vi "ESA-C Set Voltage.vi"(2 "Voltage":dbl format="%.2f", 3 "Axis":i32, 4 "Drive Connection Settings":T1={"Objective GPIB-Port"=4, "Stage GPIB-Port"=4, "Drive Selector"=0, "Drive Velocity (V/s)"=5.0} {"Drive Velocity (V/s)" min=10.0 max=160.0 step=0.1 format="%.1f"; "Drive Selector" items=["Obj.", "Stage"]; "Stage GPIB-Port" min=1 max=20 step=1 format="%#.0f"; "Objective GPIB-Port" min=1 max=20 step=1 format="%#.0f"}) -> ()   [LabVIEW 2010]
uses:
  TypeDefs/ESA-C Connection Settings.ctl
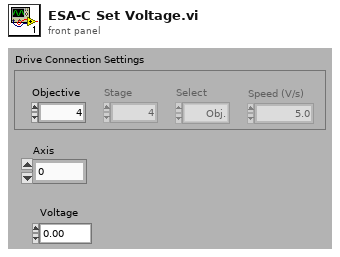
[diagram p1: front panel]
types:
  T1 = typedef "ESA-C Connection Settings.ctl" = cluster{"Objective GPIB-Port":i32, "Stage GPIB-Port":i32, "Drive Selector":u16, "Drive Velocity (V/s)":dbl}
  T2 = typedef "ESA-C Current Values.ctl" = cluster{"Voltages":cluster{"Drive X Voltage":dbl, "Drive Y Voltage":dbl, "Drive Z Voltage":dbl}, "Position":cluster{"Drive X Position":dbl, "Drive Y Position":dbl, "Drive Z Position":dbl}}
  T3 = cluster{"Drive X Voltage":dbl, "Drive Y Voltage":dbl, "Drive Z Voltage":dbl}
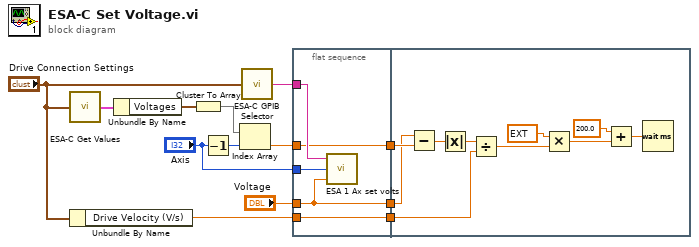
[diagram p0: block diagram]
diagram:
  n1 = call "ESA-C Get Values.vi"("Drive Connection Settings"="Drive Connection Settings") -> ("Drive Current Values"=w7:T2)
  n2 = Unbundle By Name("Drive Connection Settings") -> ("Drive Velocity (V/s)"=w3:dbl)
  n3 = Unbundle By Name(w7) -> ("Voltages"=w8:T3)
  n4 = Cluster To Array(cluster=w8) -> (array=w10:dbl[])
  n5 = Decrement(x="Axis") -> (x-1=w12:i32)
  n6 = Index Array(array=w10, index=w12) -> (element=w13:dbl)
  n7 = call "ESA-C GPIB Selector.vi"("Drive Connection Settings"="Drive Connection Settings") -> ("String"=w5:string)
  n8 = flat-sequence {
    tunnel: w5 -> [w18]
    tunnel: "Axis" -> [w17]
    tunnel: "Voltage" -> [w14]
    tunnel: w13 -> [w15]
    tunnel: [w16] -> w4
    tunnel: w3 -> [w16]
    tunnel: [w15] -> w2
    tunnel: [w14] -> w1
    tunnel: w4 -> [w23]
    tunnel: w2 -> [w20]
    tunnel: w1 -> [w19]
    frame #0 {
      n9 = call "ESA 1 Ax set volts.vi"("Voltage"=w14, "Axis"=w17, "GPIB Add"=w18) -> ()
    }
    frame #1 {
      n10 = Subtract(x=w19, y=w20) -> (x-y=w21:dbl)
      n11 = Absolute Value(x=w21) -> (abs(x)=w22:dbl)
      n12 = Divide(x=w22, y=w23) -> (x/y=w28:dbl)
      n13 = Multiply(x=ext 1000.0, y=w28) -> (x*y=w24:ext)
      n14 = Add(x=200.0, y=w24) -> (x+y=w25:ext)
      n15 = Wait (ms)(milliseconds to wait=w25) -> ()  [unwired: 1 out]
    }
  }
